vi "Write Inlet Temp.vi"(0 "Line":tag="Dev1/port0/line0:7", 5 "Outlet Temp":dbl, 9 "Product":T1=enum."LCP3", 11 "Error In":errorcluster) -> (15 "Error Out":errorcluster)   [LabVIEW 2014]
doc: "This VI generates a static analog voltage output on the line you specify."
uses:
  type defs/Product Type.ctl
  <vilib>/DAQmx/create/channels.llb/DAQmx Create Channel (AO-Voltage-Basic).vi
  <vilib>/DAQmx/write.llb/DAQmx Write (Analog DBL 1Chan 1Samp).vi
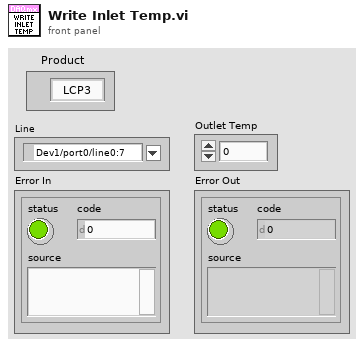
[diagram p1: front panel]
types:
  T1 = typedef "Product Type.ctl" = enum16{"Hawk", "LCP3", "2015 VA"}
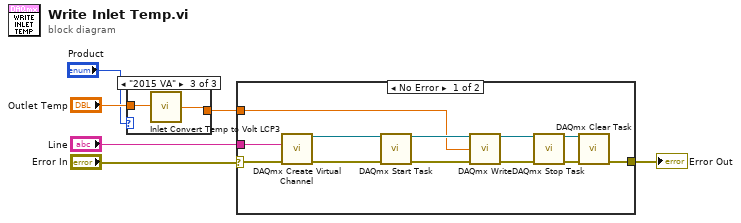
[diagram p0: block diagram]
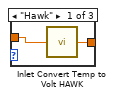
[diagram p2: hidden frame]
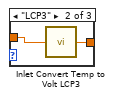
[diagram p3: hidden frame]
diagram:
  n1 = case shown="\"2015 VA\"" "Product" {
    tunnel: [w8 w10 w12] -> w2
    tunnel: "Outlet Temp" -> [w7 w9 w11]
    frame "Hawk" {
      n2 = call "Inlet Convert Temp to Volt HAWK.vi"("Inlet Temperature"=w7) -> ("Inlet Voltage"=w8:dbl)
    }
    frame "LCP3" {
      n3 = call "Inlet Convert Temp to Volt LCP3.vi"("Inlet Temperature"=w9) -> ("Inlet Voltage"=w10:dbl)
    }
    frame "2015 VA" {
      n4 = call "Inlet Convert Temp to Volt LCP3.vi"("Inlet Temperature"=w11) -> ("Inlet Voltage"=w12:dbl)
    }
  }
  n5 = case shown="No Error" "Error In" {
    selector: "Error In" -> [w16 w25]
    tunnel: "Line" -> [w15 _]
    tunnel: [w14 w25] -> w4
    tunnel: w2 -> [w13 _]
    frame No Error {
      n6 = call-poly <vilib>:"DAQmx Create Virtual Channel.vi"("physical channels"=w15, "error in"=w16) -> ("task out"=w21:refnum<k21>, "error out"=w22:errorcluster)  [unwired: 12 in]
      n7 = call <vilib>:"DAQmx Start Task.vi"("task/channels in"=w21, "error in"=w22) -> ("task out"=w24:refnum<k21>, "error out"=w23:errorcluster)  [unwired: 12 in]
      n8 = call-poly <vilib>:"DAQmx Write.vi"("task/channels in"=w24, "data"=w13, "error in"=w23) -> ("task out"=w18:refnum<k21>, "error out"=w17:errorcluster)  [unwired: 10 in, 1 out]
      n9 = call <vilib>:"DAQmx Stop Task.vi"("task/channels in"=w18, "error in"=w17) -> ("task out"=w20:refnum<k21>, "error out"=w19:errorcluster)  [unwired: 12 in]
      n10 = call <vilib>:"DAQmx Clear Task.vi"("task in"=w20, "error in"=w19) -> ("error out"=w14:errorcluster)  [unwired: 13 in]
    }
    frame Error {
    }
  }
  "Error Out" <- w4
